vi "Serial Read for Arduino with Control.vi"() -> ()   [LabVIEW 2024]
doc: "This example performs writes and reads on a serial port, as directed by the user. You can press the Write and Read buttons, and change the Read Count, while the example is running.\n\nThe parameters set for the serial port must match the parameters of the connected instrument or device. In this example, the Read Count parameter specifies the number of bytes that the serial port reads. If there were more bytes at the port than the specified number, those bytes would not be read. If there were less bytes at the port than the specified number, you would receive a timeout error.\n\nThis example expands upon the flow control options for XON and XOFF, allowing the user to choose those control characters. Also, the user can enable or disable a termination character. Some devices require a termination character in order to identify the end of command strings. Some devices send a termination character to signify the end of data to be read. This example shows how you can end the Read operation once a termination character is detected in the buffer and/or append a termination character at the end of the Write data."
uses:
  support/Serial - Settings.ctl
  <vilib>/Instr/_visa.llb/VISA Flush IO Buffer Mask.ctl
  <vilib>/Instr/_visa.llb/VISA Configure Serial Port (Instr).vi
panel:
  out "Froce Chart":dbl[][](graph)
  out "Past Time(Sec)":dbl
  out "Cantilever Chart":dbl[][](graph)
  in  "dt for Sampling (600Hz)":dbl=0.00166
  out "Filename Out":path
  out "Data Writing":bool caption="Saving Data"
  in  "Data Format":enum32{"Foece Mode", "Raw Mode"}(radio)=enum."Raw Mode"
  in  "Zero Reset":bool
  in  "Termination Character":u8=10 format="%.0x"
  in  "End Write on \nTermination Character?":bool=TRUE
  in  "Stop Measurment":bool
  in  "Serial Settings":T1={"baud rate"=115200, "data bits"=8, "parity"=enum."None", "stop bits"=10, "flow control"=0} {"flow control" items=["None"=0, "XON/XOFF"=1, "RTS/CTS"=2, "DTR/DSR"=4]; "stop bits" items=["1.0"=10, "1.5"=15, "2.0"=20]; "data bits" min=5 max=8 step=1; "baud rate" items=["75"=75, "110"=110, "134"=134, "150"=150, "300"=300, "600"=600, "1200"=1200, "1800"=1800, "2400"=2400, "4800"=4800, "7200"=7200, "9600"=9600, "14400"=14400, "19200"=19200, "28800"=28800, "38400"=38400, "56000"=56000, "57600"=57600, "115200"=115200, "128000"=128000, "230400"=230400]}
  in  "End Read on \nTermination Character?":bool=TRUE
  in  "VISA resource name":refnum<visa-resource-name>="COM1"
  # "Overview: Serial Based Data Viewer\n\nBefore Start VI \n1: Set Serial Port as Arduino Prot\n2: Select data format ( Force or Cantilever Raw)\n3: Start VI"
  # "While Operation\n1: VI asks save measirement on file as LVM format\n    If you do not need save, just cacel the dialog.\n2: If you need to switch data mode, just clock    Force or Raw.\n3: If you need to reset offcet, click zero offset."
  # "0xA is equivalent to a '\\n' character, which is a line feed."
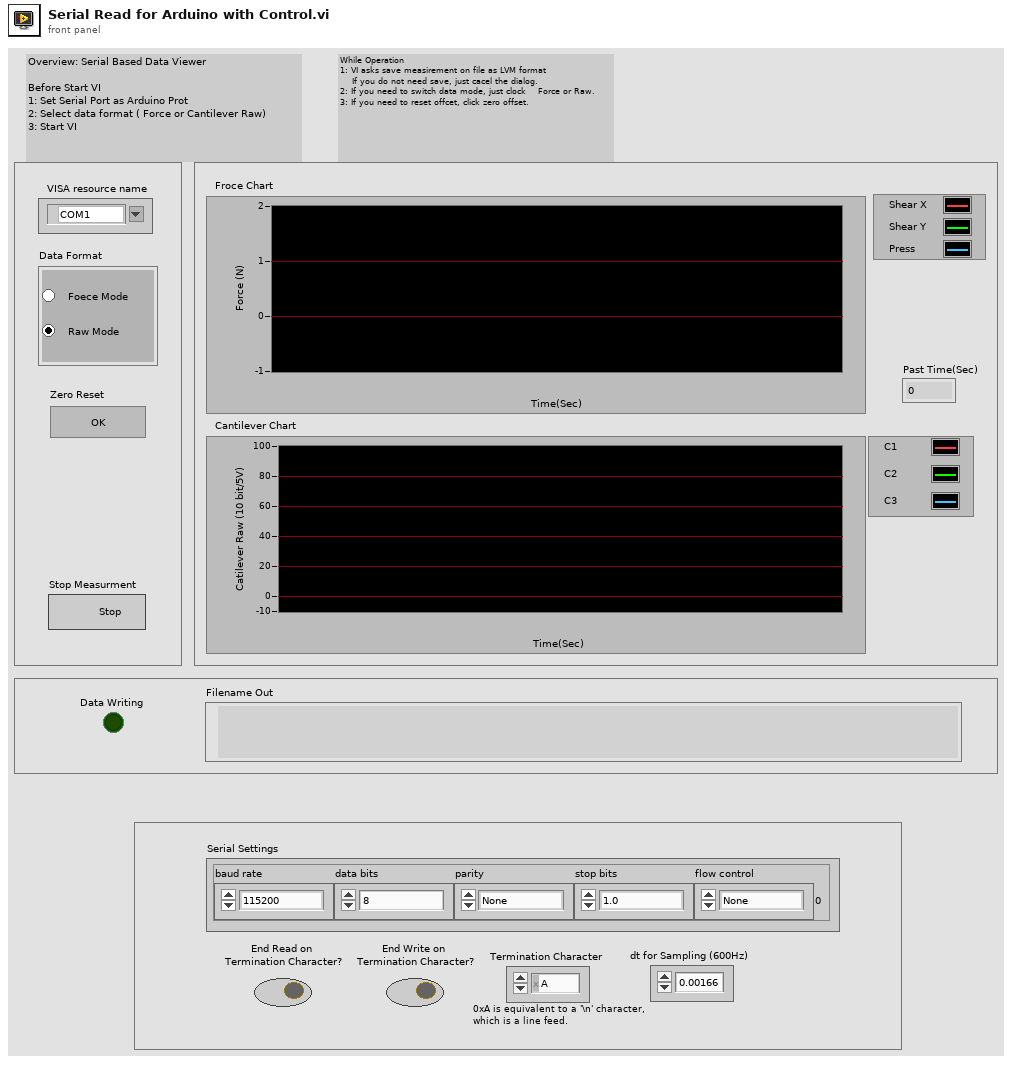
[diagram p1: front panel]
types:
  T1 = typedef "Serial - Settings.ctl" = cluster{"baud rate":u32, "data bits":u16, "parity":enum16{"None", "Odd", "Even", "Mark", "Space"}, "stop bits":u16, "flow control":u16}
  T2 = typedef "VISA Flush IO Buffer Mask.ctl" = u16
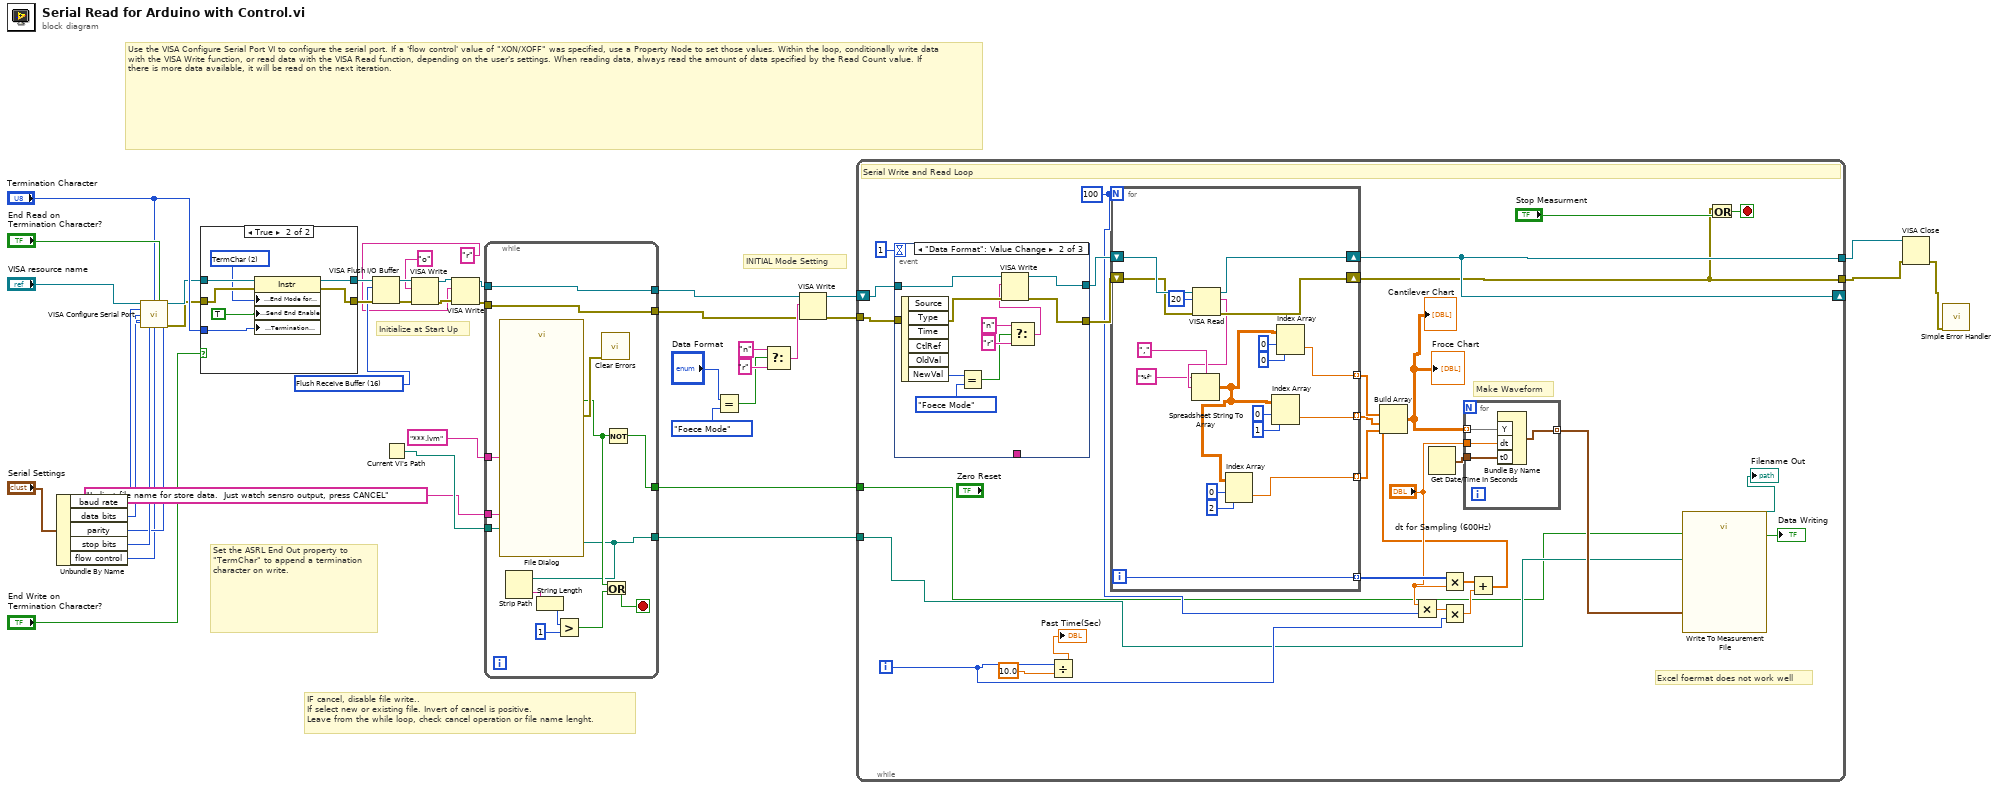
[diagram p0: block diagram]
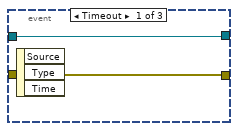
[diagram p3: hidden frame]
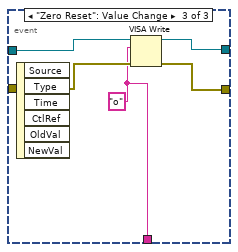
[diagram p4: hidden frame]
diagram:
  w24 = T2 16 items=["Flush Receive Buffer"=16, "Write Transmit Buffer to Device"=32, "Flush Receive Buffer (No I/O)"=64, "Flush Transmit Buffer"=128] ("Mask")
  # "INITIAL Mode Setting"
  # "IF cancel, disable file write..\nIf select new or existing file. Invert of cancel is positive.\nLeave from the while loop, check cancel operation or file name lenght."
  # "Initialize at Start Up"
  # "Set the ASRL End Out property to \"TermChar\" to append a termination character on write."
  # "Use the VISA Configure Serial Port VI to configure the serial port. If a 'flow control' value of \"XON/XOFF\" was specified, use a Property Node to set those values. Within the loop, conditionally write data with the VISA Write function, or read data with the VISA Read function, depending on the user's settings. When reading data, always read the amount of data specified by the Read Count value. If there is more data available, it will be read on the next iteration."
  n1 = Unbundle By Name("Serial Settings") -> ("baud rate"=w37:u32, "data bits"=w38:u16, "parity"=w39:enum16{"None", "Odd", "Even", "Mark", "Space"}, "stop bits"=w40:u16, "flow control"=w34:u16)
  n2 = call-poly "VISA Configure Serial Port"("VISA resource name"="VISA resource name", "termination char\n(0xA = '\\n' = LF)"="Termination Character", "Enable Termination\nChar (T)"="End Read on \nTermination Character?", "baud rate (9600)"=w37, "data bits (8)"=w38, "parity (0:none)"=w39, "stop bits (10: 1 bit)"=w40, "flow control (0:none)"=w34) -> ("VISA resource name out"=w31:refnum<visa-resource-name>, "error out"=w30:errorcluster)  [unwired: 2 in, 4 out]
  n3 = case shown="True" "End Write on \nTermination Character?" {
    tunnel: w31 -> [w42 w50]
    tunnel: w30 -> [w43 w49]
    tunnel: [w42 w48] -> w26
    tunnel: [w43 w47] -> w25
    tunnel: "Termination Character" -> [_ w45]
    frame False {
    }
    frame True {
      w46 = u16 2 items=["None", "LastBit", "TermChar", "Break"] ("Serial Settings:Serial End Mode for Writes")
      n4 = property class="Instr"(reference=w50, error in=w49, "Serial Settings:End Mode for Writes"=w46, "Message Based Settings:Send End Enable"=TRUE, "Message Based Settings:Termination Character"=w45) -> (reference out=w48:refnum<visa-resource-name>, error out=w47:errorcluster)
    }
  }
  n5 = VISA Flush I/O Buffer(VISA resource name=w26, mask (16)=w24, error in (no error)=w25) -> (VISA resource name out=w23:refnum<visa-resource-name>, error out=w22:errorcluster)
  n6 = Current VI's Path() -> (path=w13:path)
  n7 = VISA Write(VISA resource name=w23, write buffer="o", error in (no error)=w22) -> (VISA resource name out=w20:refnum<visa-resource-name>, error out=w19:errorcluster)  [unwired: 1 out]
  n8 = VISA Write(VISA resource name=w20, write buffer="r", error in (no error)=w19) -> (VISA resource name out=w17:refnum<visa-resource-name>, error out=w16:errorcluster)  [unwired: 1 out]
  n9 = while {
    tunnel: [w64] -> w5
    tunnel: w17 -> [w64]
    tunnel: [w63] -> w4
    tunnel: w16 -> [w63]
    tunnel: [w55] -> w15
    tunnel: [w61] -> w14
    tunnel: w13 -> [w60]
    tunnel: "Indicat file name for store data.  Just watch sensro output, press CANCEL" ("prompt") -> [w57]
    tunnel: "***.lvm" ("default name") -> [w51]
    stop <- w58 stop-if-true
    n10 = call "File Dialog"("start path"=w60, "prompt"=w57, "default name"=w51) -> ("selected path"=w55:path, "cancelled"=w59:bool, "error out"=w62:errorcluster)  [unwired: 9 in, 1 out]
    n11 = Strip Path(path=w55) -> (name=w56:string)  [unwired: 1 out]
    n12 = String Length(string=w56) -> (length=w54:i32)
    n13 = Greater?(x=w54, y=1) -> (0:w52:bool)
    n14 = call <vilib>:"Clear Errors.vi"("error in (no error)"=w62) -> ()  [unwired: 5 in, 2 out]
    n15 = Or(x=w59, y=w52) -> (x .or. y?=w58:bool)
    n16 = Not(x=w59) -> (.not. x?=w61:bool)
  }
  n17 = Equal?(x="Data Format", y=enum16{"Foece Mode", "Raw Mode", ""}."Foece Mode") -> (x = y?=w2:bool)
  n18 = Select(t="n", s=w2, f="r") -> (s? t:f=w8:string)
  n19 = VISA Write(VISA resource name=w5, write buffer=w8, error in (no error)=w4) -> (VISA resource name out=w7:refnum<visa-resource-name>, error out=w6:errorcluster)  [unwired: 1 out]
  n20 = while {
    shift-right: [w91] -> _
    shift-left: w7 -> [w88]
    tunnel: w6 -> [w89]
    tunnel: [w90] -> w29
    tunnel: [w91] -> w28
    tunnel: w15 -> [w66]
    tunnel: w14 -> [w65]
    i -> [w71]
    stop <- w93 stop-if-true
    w74 = 100
    # "Excel foermat does not work well"
    # "Make Waveform"
    # "Serial Write and Read Loop"
    n21 = event shown="[1] \"Data Format\": Value Change" {
      selector: _ -> [_ _ _]
      dyn-events: _ -> [_ _ _]
      timeout: 1 -> [_ _ _]
      tunnel: w89 -> [w98 w108 w114]
      tunnel: w88 -> [w99 w109 w113]
      tunnel: [w99 w106 w112] -> w87
      tunnel: [w98 w107 w111] -> w86
      tunnel: [_ _ w110] -> _
      event Timeout {
        n22 = event-data() -> ()  [unwired: 1 in, 3 out]
      }
      event "Data Format": Value Change {
        n23 = event-data() -> ("NewVal"=w104:enum32{"Foece Mode", "Raw Mode"})  [unwired: 1 in, 5 out]
        n24 = Equal?(x=w104, y=enum16{"Foece Mode", "Raw Mode", ""}."Foece Mode") -> (x = y?=w101:bool)
        n25 = Select(t="n", s=w101, f="r") -> (s? t:f=w100:string)
        n26 = VISA Write(VISA resource name=w109, write buffer=w100, error in (no error)=w108) -> (VISA resource name out=w106:refnum<visa-resource-name>, error out=w107:errorcluster)  [unwired: 1 out]
      }
      event "Zero Reset": Value Change {
        w110 = "o" ("write buffer")
        n27 = event-data() -> ()  [unwired: 1 in, 6 out]
        n28 = VISA Write(VISA resource name=w113, write buffer=w110, error in (no error)=w114) -> (VISA resource name out=w112:refnum<visa-resource-name>, error out=w111:errorcluster)  [unwired: 1 out]
      }
    }
    n29 = Divide(x=w71, y=10.0 ("x")) -> (x/y=→"Past Time(Sec)":dbl)
    n30 = for {
      N: w74 -> [_]
      shift-right: [w130] -> w91
      shift-left: w87 -> [w133]
      shift-right: [w131] -> w90
      shift-left: w86 -> [w132]
      tunnel: [w122] -> w76 mode=indexing
      tunnel: [w121] -> w77 mode=indexing
      tunnel: [w117] -> w75 mode=indexing
      tunnel: [w115] -> w78 mode=indexing
      i -> [w115]
      n31 = VISA Read(VISA resource name=w133, byte count=u32 20, error in (no error)=w132) -> (VISA resource name out=w130:refnum<visa-resource-name>, read buffer=w124:string, error out=w131:errorcluster)  [unwired: 1 out]
      n32 = Spreadsheet String To Array(delimiter (Tab)=",", format string="%f", spreadsheet string=w124) -> (array=w118:dbl[][])  [unwired: 1 in]
      n33 = Index Array(array=w118, index (row)=0, index (col)=2 ("disabled index (col)")) -> (element=w117:dbl)
      n34 = Index Array(array=w118, index (row)=0, index (col)=1 ("disabled index (col)")) -> (element=w122:dbl)
      n35 = Index Array(array=w118, index (row)=0, index (col)=0 ("disabled index (col)")) -> (element=w121:dbl)
    }
    n36 = Multiply(x="dt for Sampling (600Hz)", y=w74) -> (x*y=w70:dbl)
    n37 = Get Date/Time In Seconds() -> (seconds since 1Jan1904=w79:timestamp)
    n38 = Multiply(x=w78, y="dt for Sampling (600Hz)") -> (x*y=w69:dbl[])
    n39 = Multiply(x=w70, y=w71) -> (x*y=w72:dbl)
    n40 = Add(x=w69, y=w72) -> (x+y=w68:dbl[])
    n41 = Build Array(w68, w77, w76, w75) -> (w81:dbl[][])
    "Cantilever Chart" <- w81
    "Froce Chart" <- w81
    n42 = for {
      tunnel: w81 -> [w95] mode=indexing
      tunnel: [w97] -> w83 mode=indexing
      tunnel: "dt for Sampling (600Hz)" -> [w96]
      tunnel: w79 -> [w94]
      n43 = Bundle By Name("Y"=w95, "dt"=w96, "t0"=w94) -> (w97:waveform(dbl))  [unwired: 1 in]
    }
    n44 = call "Write To Measurement File"("Signals"=w83, "Enable"=w65, "Filename"=w66) -> ("Filename Out"=→"Filename Out":path, "Saving Data"=→"Data Writing":bool)  [unwired: 14 in, 1 out]
    n45 = Or(x=w90, y="Stop Measurment") -> (x .or. y?=w93:bool)
  }
  n46 = VISA Close(VISA resource name=w28, error in (no error)=w29) -> (error out=w27:errorcluster)
  n47 = call <vilib>:"Simple Error Handler.vi"("error in (no error)"=w27) -> ()  [unwired: 1 in, 8 out]
